vi "Date Time String difference in secs.vi"(8 "error in (no error)":errorcluster, 10 "Ending time":string, 11 "Starting time":string) -> (0 "error out":errorcluster, 1 "Total Seconds difference":u32, 2 "Ending Timestamp":timestamp, 3 "Starting Timestamp":timestamp, 4 "Minutes difference":u32, 5 "Seconds difference":dbl)   [LabVIEW 2013]
doc: "This example is used to convert a date and time string back into a timestamp."
uses:
  <vilib>/Utility/miscctls.llb/LVDateTimeRec.ctl
panel:
  out "Timestamp from Date/Time String 2":timestamp
  out "Number of Seconds 2":u64
  out "Number of Seconds":u64
  out "Timestamp from Date/Time String":timestamp
  # "Derived/Computed Values"
  # "Note: the only thing that's off is the Fractional Seconds, but that's because you don't have that information\nin the date/time string"
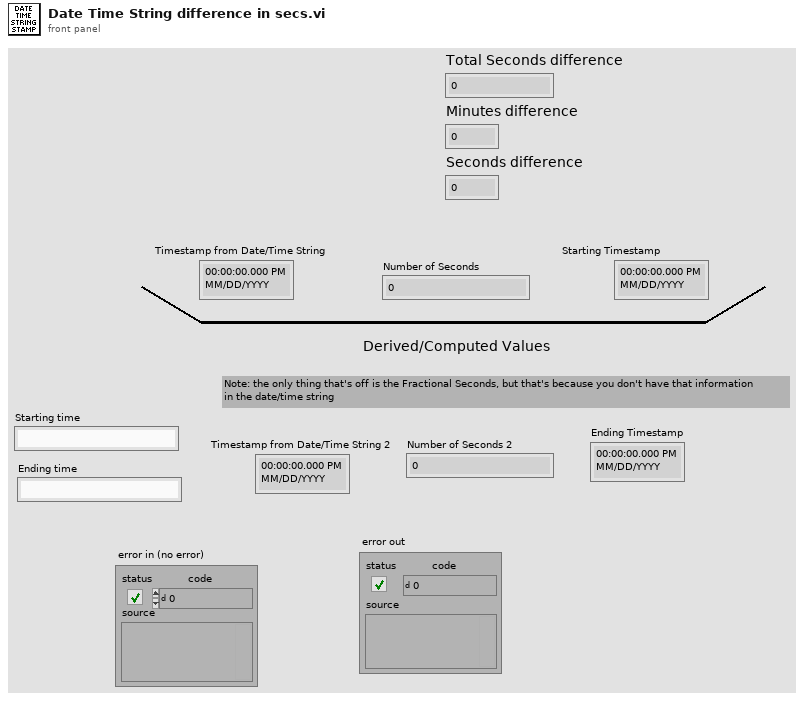
[diagram p1: front panel]
types:
  T1 = typedef "LVDateTimeRec.ctl" = cluster{"fractional second":dbl, "second":i32, "minute":i32, "hour":i32, "day of month":i32, "month":i32, "year":i32, "day of week":i32, "day of year":i32, "DST":i32}
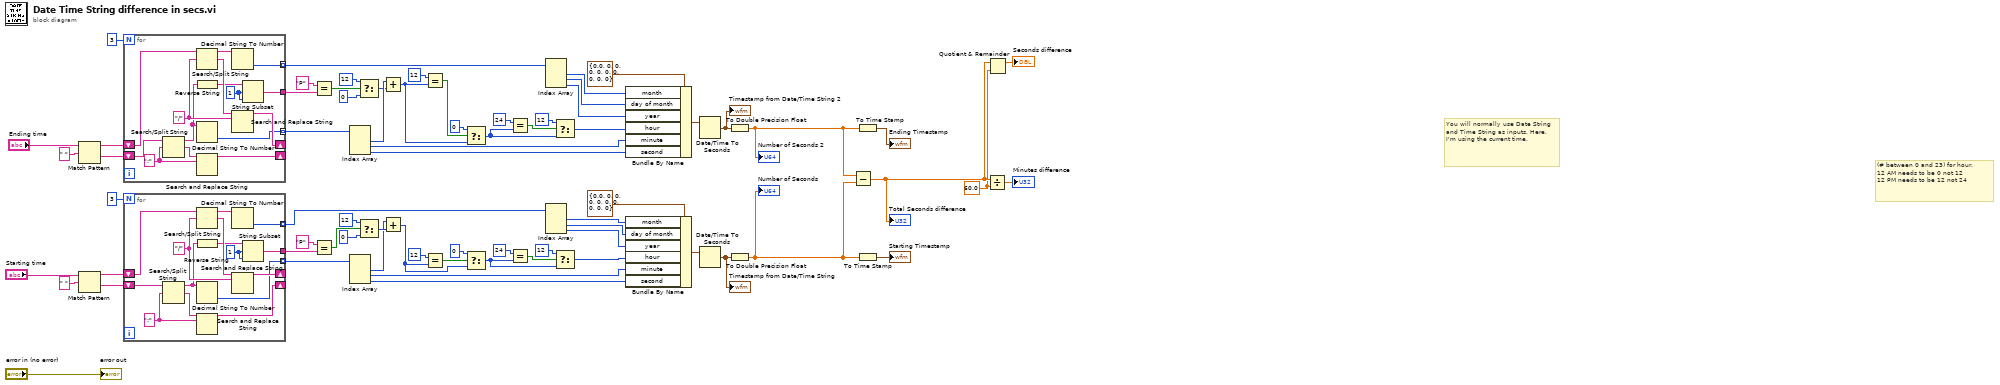
[diagram p0: block diagram]
diagram:
  w2 = 60.0 ("y")
  # "You will normally use Date String and Time String as inputs. Here, I'm using the current time."
  # "(# between 0 and 23) for hour.\n12 AM needs to be 0 not 12\n12 PM needs to be 12 not 24"
  n1 = Match Pattern(string="Ending time", regular expression=" ") -> (before substring=w37:string, after substring=w38:string)  [unwired: 1 in, 2 out]
  n2 = Match Pattern(string="Starting time", regular expression=" ") -> (before substring=w41:string, after substring=w40:string)  [unwired: 1 in, 2 out]
  n3 = for {
    N: 3 -> [_]
    shift-right: [w84] -> _
    shift-left: w37 -> [w85]
    tunnel: [w82] -> w18 mode=indexing
    shift-right: [w81] -> _
    shift-left: w38 -> [w77]
    tunnel: [w78] -> w11 mode=indexing
    tunnel: [w72] -> w9
    w73 = 1 ("offset (0)")
    w79 = ":" ("search string/char (-)")
    w80 = "/" ("search string/char (-)")
    n4 = Search/Split String(string=w77, search string/char (-)=w79) -> (substring before match=w75:string, match + rest of string=w76:string)  [unwired: 1 in, 1 out]
    n5 = Search/Split String(string=w85, search string/char (-)=w80) -> (substring before match=w83:string, match + rest of string=w86:string)  [unwired: 1 in, 1 out]
    n6 = Reverse String(1:w75) -> (0:w74:string)
    n7 = Decimal String To Number(string=w75) -> (number=w78:i32)  [unwired: 2 in, 1 out]
    n8 = Search and Replace String(input string=w76, search string=w79) -> (result string=w81:string)  [unwired: 6 in, 3 out]
    n9 = Decimal String To Number(string=w83) -> (number=w82:i32)  [unwired: 2 in, 1 out]
    n10 = Search and Replace String(input string=w86, search string=w80) -> (result string=w84:string)  [unwired: 6 in, 3 out]
    n11 = String Subset(string=w74, offset (0)=w73, length (rest)=w73) -> (substring=w72:string)
  }
  n12 = for {
    N: 3 -> [_]
    shift-right: [w99] -> _
    shift-left: w41 -> [w100]
    tunnel: [w97] -> w61 mode=indexing
    shift-right: [w96] -> _
    shift-left: w40 -> [w92]
    tunnel: [w93] -> w68 mode=indexing
    tunnel: [w87] -> w70
    w88 = 1 ("offset (0)")
    w94 = ":" ("search string/char (-)")
    w95 = "/" ("search string/char (-)")
    n13 = Search/Split String(string=w92, search string/char (-)=w94) -> (substring before match=w90:string, match + rest of string=w91:string)  [unwired: 1 in, 1 out]
    n14 = Search/Split String(string=w100, search string/char (-)=w95) -> (substring before match=w98:string, match + rest of string=w101:string)  [unwired: 1 in, 1 out]
    n15 = Reverse String(1:w90) -> (0:w89:string)
    n16 = Decimal String To Number(string=w90) -> (number=w93:i32)  [unwired: 2 in, 1 out]
    n17 = Search and Replace String(input string=w91, search string=w94) -> (result string=w96:string)  [unwired: 6 in, 3 out]
    n18 = Decimal String To Number(string=w98) -> (number=w97:i32)  [unwired: 2 in, 1 out]
    n19 = Search and Replace String(input string=w101, search string=w95) -> (result string=w99:string)  [unwired: 6 in, 3 out]
    n20 = String Subset(string=w89, offset (0)=w88, length (rest)=w88) -> (substring=w87:string)
  }
  n21 = Equal?(x="P", y=w9) -> (x = y?=w12:bool)
  n22 = Equal?(x="P", y=w70) -> (x = y?=w67:bool)
  n23 = Index Array(array=w11) -> (element #1=w16:i32, element #2=w22:i32, element #3=w23:i32)  [unwired: 3 in]
  n24 = Index Array(array=w68) -> (element #1=w63:i32, element #2=w57:i32, element #3=w56:i32)  [unwired: 3 in]
  n25 = Select(t=12 ("index"), s=w12, f=0 ("index")) -> (s? t:f=w15:i32)
  n26 = Select(t=12 ("index"), s=w67, f=0 ("index")) -> (s? t:f=w64:i32)
  n27 = Add(x=w16, y=w15) -> (x+y=w29:i32)
  n28 = Add(x=w63, y=w64) -> (x+y=w50:i32)
  n29 = Equal?(x=12 ("y"), y=w29) -> (x = y?=w27:bool)
  n30 = Equal?(x=12 ("y"), y=w50) -> (x = y?=w52:bool)
  n31 = Select(t=0, s=w27, f=w29) -> (s? t:f=w32:i32)
  n32 = Select(t=0, s=w52, f=w50) -> (s? t:f=w47:i32)
  n33 = Equal?(x=24 ("y"), y=w32) -> (x = y?=w25:bool)
  n34 = Equal?(x=24 ("y"), y=w47) -> (x = y?=w54:bool)
  n35 = Index Array(array=w18) -> (element #1=w19:i32, element #2=w20:i32, element #3=w21:i32)  [unwired: 3 in]
  n36 = Index Array(array=w61) -> (element #1=w60:i32, element #2=w59:i32, element #3=w58:i32)  [unwired: 3 in]
  n37 = Select(t=12 ("index"), s=w25, f=w32) -> (s? t:f=w33:i32)
  n38 = Select(t=12 ("index"), s=w54, f=w47) -> (s? t:f=w46:i32)
  n39 = Bundle By Name(cluster=T1 {"fractional second"=0.0, "second"=0, "minute"=0, "hour"=0, "day of month"=0, "month"=0, "year"=0, "day of week"=0, "day of year"=0, "DST"=0} ("date time rec"), "month"=w19, "day of month"=w20, "year"=w21, "hour"=w33, "minute"=w22, "second"=w23) -> (w24:T1)
  n40 = Bundle By Name(cluster=T1 {"fractional second"=0.0, "second"=0, "minute"=0, "hour"=0, "day of month"=0, "month"=0, "year"=0, "day of week"=0, "day of year"=0, "DST"=0} ("date time rec"), "month"=w60, "day of month"=w59, "year"=w58, "hour"=w46, "minute"=w57, "second"=w56) -> (w55:T1)
  n41 = Date/Time To Seconds(2:w24) -> (0:w34:timestamp)  [unwired: 1 in]
  "Timestamp from Date/Time String 2" <- w34
  n42 = Date/Time To Seconds(2:w55) -> (0:w45:timestamp)  [unwired: 1 in]
  "Timestamp from Date/Time String" <- w45
  n43 = To Double Precision Float(number=w34) -> (double precision float=w6:dbl)
  "Number of Seconds 2" <- w6
  n44 = To Double Precision Float(number=w45) -> (double precision float=w5:dbl)
  "Number of Seconds" <- w5
  n45 = Subtract(x=w6, y=w5) -> (x-y=w3:dbl)
  "Total Seconds difference" <- w3
  n46 = To Time Stamp(1:w6) -> (0:→"Ending Timestamp":timestamp)
  n47 = To Time Stamp(1:w5) -> (0:→"Starting Timestamp":timestamp)
  n48 = Divide(x=w3, y=w2) -> (x/y=→"Minutes difference":dbl)
  n49 = Quotient & Remainder(x=w3, y=w2) -> (x-y*floor(x/y)=→"Seconds difference":dbl)  [unwired: 1 out]
  "error out" <- "error in (no error)"
